vi "XY Graph Find Plot CC Shift.vi"(4 "Half Width (Points)":i32=5, 6 "polynomial order":i32=3, 7 "normalization":enum32{"none", "unbiased", "biased"}(ring)=enum."unbiased", 8 "Error In":errorcluster, 9 "Ref Array":dbl[](array[numeric]), 10 "Y Array":dbl[](array[numeric]), 11 "X Array":dbl[](array[numeric])) -> (0 "Error Out":errorcluster, 1 "Shift (Index Unit)":dbl, 3 "Shift":dbl)   [LabVIEW 2021, in "XY Graph Add-Ons.lvlib"]
uses:
  XY Graph Add-Ons.lvlib
  <vilib>/Utility/error.llb/DialogType.ctl
  <vilib>/Analysis/6fits.llb/Curve Fitting Criteria.ctl
  <vilib>/Analysis/2dsp.llb/1D Cross Correlation (DBL).vi
  <vilib>/Analysis/NI_AALPro.lvlib
  <vilib>/gmath/NI_Gmath.lvlib
  Strings/Strings.lvlib
  Formula/Formula.lvlib
  Error/Error.lvlib
panel:
  out "XY Graph":cluster{dbl[], "Rxy":dbl[]}[](graph)
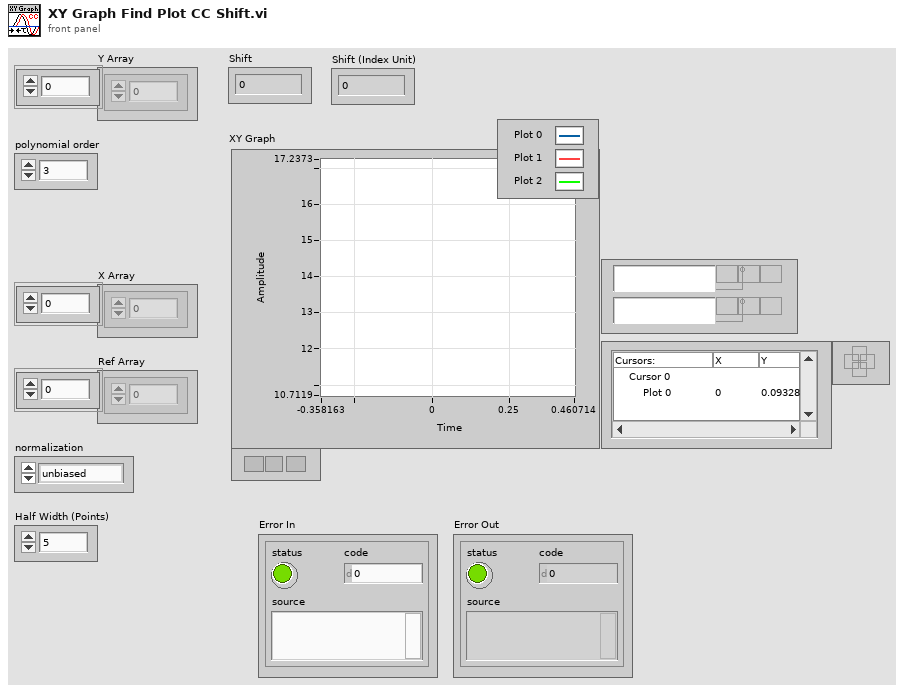
[diagram p1: front panel]
types:
  T1 = typedef "DialogType.ctl" = u16
  T2 = typedef "NI_AALPro.lvlib/Curve Fitting Criteria.ctl" = u16
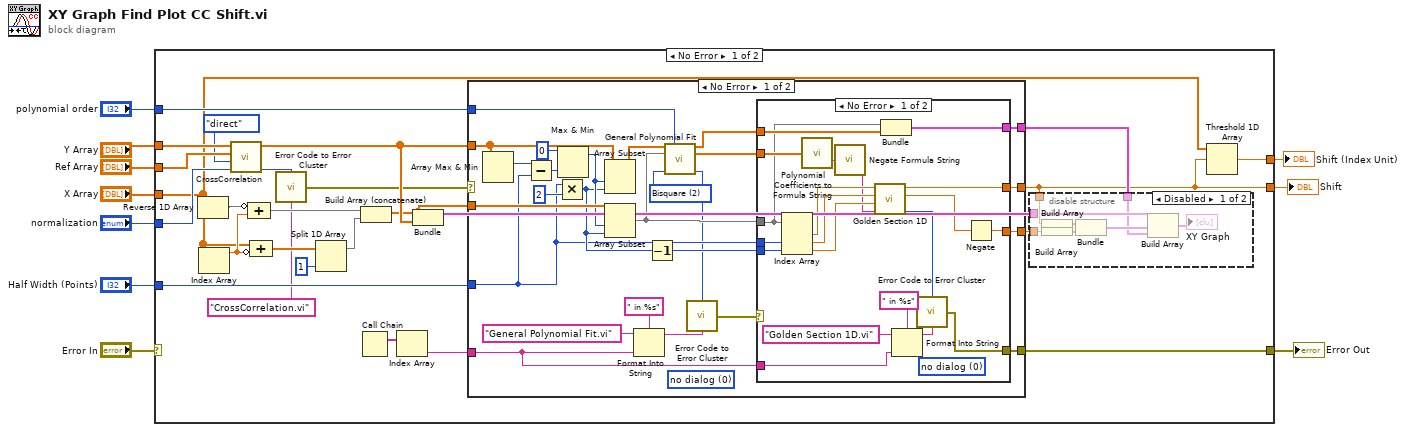
[diagram p0: block diagram]
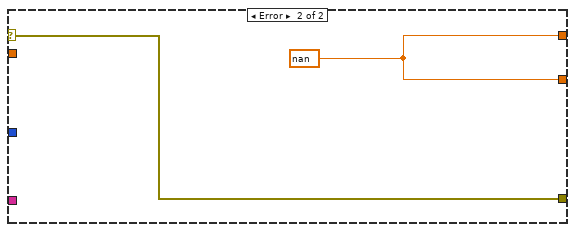
[diagram p4: hidden frame]
diagram:
  n1 = case shown="No Error" "Error In" {
    selector: "Error In" -> [_ w94]
    tunnel: "normalization" -> [w36 _]
    tunnel: "polynomial order" -> [w35 _]
    tunnel: "Half Width (Points)" -> [w34 _]
    tunnel: [w18 _] -> w7
    tunnel: "X Array" -> [w17 _]
    tunnel: "Ref Array" -> [w33 _]
    tunnel: "Y Array" -> [w32 _]
    tunnel: [w19 w94] -> w2
    tunnel: [w16 _] -> w1
    frame No Error {
      n2 = Reverse 1D Array(array=w17) -> (reversed array=w29:dbl[])
      n3 = Index Array(array=w17) -> (element=w28:dbl)  [unwired: 1 in]
      n4 = call-poly <vilib>:"CrossCorrelation.vi"("normalization"=w36, "algorithm"=enum32{"direct", "frequency domain"}."direct", "Y"=w33, "X"=w32) -> ("error"=w13:i32, "Rxy"=w24:dbl[])  [unwired: 6 in]
      n5 = Compound Arithmetic op=ADD(invert w29, w28) -> (w25:dbl[])
      n6 = Compound Arithmetic op=ADD(w17, invert w28) -> (w30:dbl[])
      n7 = call "Error Code to Error Cluster.vi"("Error Code"=w13, "Error Source"="CrossCorrelation.vi" ("error source (\" \")")) -> ("Error Out"=w11:errorcluster)  [unwired: 13 in]
      n8 = Split 1D Array(array=w30, index=1) -> (second subarray=w27:dbl[])  [unwired: 1 out]
      n9 = Call Chain() -> (call chain=w15:string[])
      n10 = Build Array (concatenate)(w25, w27) -> (w23:dbl[])
      n11 = Index Array(array=w15) -> (element=w14:string)  [unwired: 1 in]
      n12 = Bundle(w23, "Rxy"=w24) -> (w21:cluster{dbl[], "Rxy":dbl[]})  [unwired: 1 in]
      n13 = case shown="No Error" w11 {
        selector: w11 -> [_ w92]
        tunnel: w24 -> [w66 _]
        tunnel: w23 -> [w64 _]
        tunnel: [w60 w93] -> w18
        tunnel: w34 -> [w56 _]
        tunnel: [w52 w93] -> w22
        tunnel: w35 -> [w61 _]
        tunnel: [w53 _] -> w20
        tunnel: [w50 w92] -> w19
        tunnel: w14 -> [w48 _]
        frame No Error {
          (unwired) T1 0 items=["no dialog", "OK message", "continue or stop message", "OK message + warnings", "continue/stop + warnings"] ("type of dialog (OK msg:1)")
          w62 = T2 2 items=["Least Square", "Least Absolute Residual", "Bisquare"] ("method")
          n14 = Array Max & Min(array=w66) -> (max index (indices)=w70:i32)  [unwired: 3 out]
          n15 = Subtract(x=w70, y=w56) -> (x-y=w69:i32)
          n16 = Multiply(x=w56, y=2) -> (x*y=w58:i32)
          n17 = Max & Min(x=0, y=w69) -> (max(x,y)=w63:i32)  [unwired: 1 out]
          n18 = Array Subset(array=w66, index=w63, length=w58) -> (w65:dbl[])
          n19 = Array Subset(array=w64, index=w63, length=w58) -> (w54:dbl[])
          n20 = Format Into String(format string=" in %s", initial string="General Polynomial Fit.vi" ("error source (\" \")"), w48) -> (resulting string=w46:string)  [unwired: 1 in, 1 out]
          n21 = Decrement(x=w58) -> (x-1=w57:i32)
          n22 = call <vilib>:"General Polynomial Fit.vi"("Y"=w65, "polynomial order"=w61, "X"=w54, "method"=w62) -> ("Best Polynomial Fit"=w55:dbl[], "Polynomial Coefficients"=w59:dbl[], "error"=w47:i32)  [unwired: 8 in, 1 out]
          n23 = call "Error Code to Error Cluster.vi"("Error Code"=w47, "Error Source"=w46) -> ("Error Out"=w45:errorcluster)  [unwired: 13 in]
          n24 = case shown="No Error" w45 {
            selector: w45 -> [_ w91]
            tunnel: [w90 _] -> w60
            tunnel: w59 -> [w88 _]
            tunnel: w57 -> [w85 _]
            tunnel: w56 -> [w84 _]
            tunnel: w55 -> [w81 _]
            tunnel: w54 -> [w80 _]
            tunnel: [w79 _] -> w53
            tunnel: [w77 _] -> w52
            tunnel: [w71 w91] -> w50
            tunnel: w48 -> [w74 _]
            frame No Error {
              (unwired) T1 0 items=["no dialog", "OK message", "continue or stop message", "OK message + warnings", "continue/stop + warnings"] ("type of dialog (OK msg:1)")
              n25 = Index Array(array=w80, index #2=w84, index #3=w85) -> (element #1=w86:dbl, element #2=w83:dbl, element #3=w82:dbl)  [unwired: 1 in]
              n26 = call "Polynomial Coefficients to Formula String.vi"("Polynomial Coefficients"=w88) -> ("formula"=w87:string)  [unwired: 8 in]
              n27 = call "Negate Formula String.vi"("formula"=w87) -> ("- formula"=w78:string)  [unwired: 8 in]
              n28 = call <vilib>:"Golden Section 1D.vi"("formula"=w78, "c (start)"=w82, "b (start)"=w83, "a (start)"=w86) -> ("error"=w73:i32, "f(minimum)"=w89:dbl, "minimum"=w90:dbl)  [unwired: 1 in, 1 out]
              n29 = Bundle(w80, "Best Polynomial Fit"=w81) -> (w79:cluster{dbl[], "Best Polynomial Fit":dbl[]})  [unwired: 1 in]
              n30 = Format Into String(format string=" in %s", initial string="Golden Section 1D.vi" ("error source (\" \")"), w74) -> (resulting string=w72:string)  [unwired: 1 in, 1 out]
              n31 = call "Error Code to Error Cluster.vi"("Error Code"=w73, "Error Source"=w72) -> ("Error Out"=w71:errorcluster)  [unwired: 13 in]
              n32 = Negate(x=w89) -> (-x=w77:dbl)
            }
            frame Error {
            }
          }
        }
        frame Error {
          w93 = nan ("Numeric Control")
        }
      }
      n33 = disable-structure shown="Disabled" {
        disable-tunnel: w18 -> [w44 _]
        disable-tunnel: w22 -> [w43 _]
        disable-tunnel: w21 -> [w39 _]
        disable-tunnel: w20 -> [w37 _]
        frame Disabled {
          n34 = Build Array(w44) -> (w41:dbl[])
          n35 = Build Array(w43) -> (w40:dbl[])
          n36 = Bundle(w41, w40) -> (w42:cluster{dbl[], dbl[]})  [unwired: 1 in]
          n37 = Build Array(w39, w42, w37) -> (→"XY Graph":cluster{dbl[], "Best Polynomial Fit":dbl[]}[])
        }
        frame Enabled {
        }
      }
      n38 = Threshold 1D Array(2:w18, 3:w17) -> (0:w16:dbl)  [unwired: 1 in]
    }
    frame Error {
    }
  }
  "Shift" <- w7
  "Error Out" <- w2
  "Shift (Index Unit)" <- w1
